vi "search_and_replace.vi"(8 "error in (no error)":errorcluster, 9 "configuration_to_replace":T1={"tag_name"="", "type"="<type>", "zero"=0.0, "formula"="", "points"=[]}, 10 "tag_name":string, 11 "configuration in":T1[](array[typedef])) -> (0 "error out":errorcluster, 3 "configuration out":T1[](array[typedef]))   [LabVIEW 2015, in "lv-calibration.lvlib"]
uses:
  lv-calibration.lvlib
  _controls/configuration.ctl
  _controls/type.ctl
  _controls/point.ctl
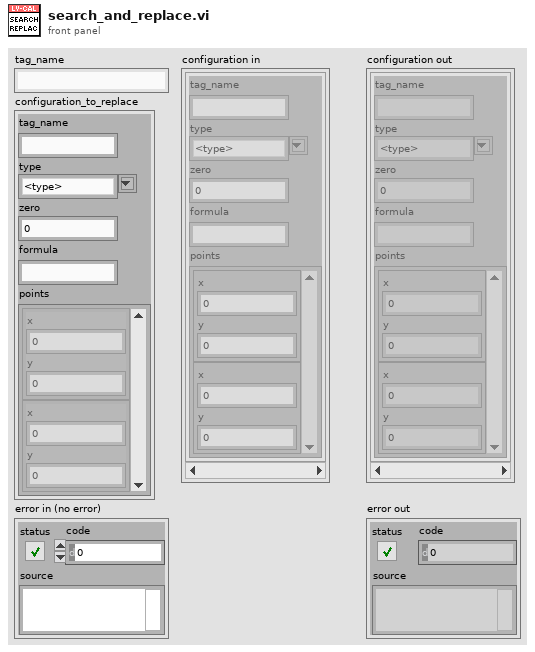
[diagram p1: front panel]
types:
  T1 = typedef "lv-calibration.lvlib/configuration.ctl" = cluster{"tag_name":string, "type":T2, "zero":dbl, "formula":string, "points":T3[]}
  T2 = typedef "lv-calibration.lvlib/type.ctl" = string
  T3 = typedef "lv-calibration.lvlib/point.ctl" = cluster{"x":dbl, "y":dbl}
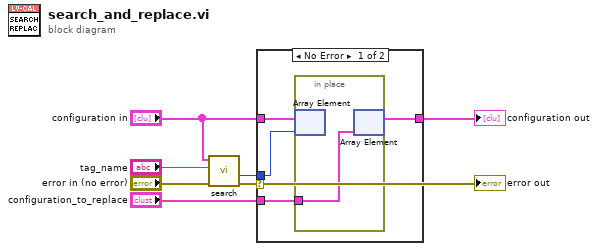
[diagram p0: block diagram]
diagram:
  n1 = call "search.vi"("error in (no error)"="error in (no error)", "tag_name"="tag_name", "configuration []"="configuration in") -> ("error out"=w1:errorcluster, "index"=w4:i32)  [unwired: 6 in, 1 out]
  "error out" <- w1
  n2 = case shown="No Error" w1 {
    tunnel: "configuration in" -> [w11 w13]
    tunnel: w4 -> [w10 _]
    tunnel: "configuration_to_replace" -> [w9 _]
    tunnel: [w8 w13] -> w2
    frame No Error {
      n3 = in-place {
        in-place-border: w9 -> [w12]
        n4 = in-place-array #1(w11, w10) -> ()  [unwired: 1 out]
        n5 = in-place-array #1(w12) -> (w8:T1[])  [unwired: 1 out]
      }
    }
    frame Error {
    }
  }
  "configuration out" <- w2
